vi "Actor Core.vi"(8 "error in":errorcluster caption="错误输入", 11 "上位机 in":refnum<class "上位机.lvclass"> caption="操作者输入") -> (0 "error out":errorcluster caption="错误输出", 3 "Actor out":refnum<class "Actor.lvclass"> caption="操作者输出")   [LabVIEW 2015, in "上位机.lvlib" / "上位机.lvclass"]
doc: "(<B>Filename</B>: Actor Framework.lvlib:Actor.lvclass:Actor Core.vi)\n\nReceives messages to the actor, reacts to them, and initiates any error handling that may shut the actor down.\n\nDescendant classes may override this VI to append parallel tasks for the actor to complete while it handles messages. Overrides use the Call Parent Method node."
uses:
  <vilib>/ActorFramework/Actor/Actor.lvclass
panel:
  in  "上位机标题":string
  out "接收内容":string
  in  "发送内容":string
  in  "发送":bool
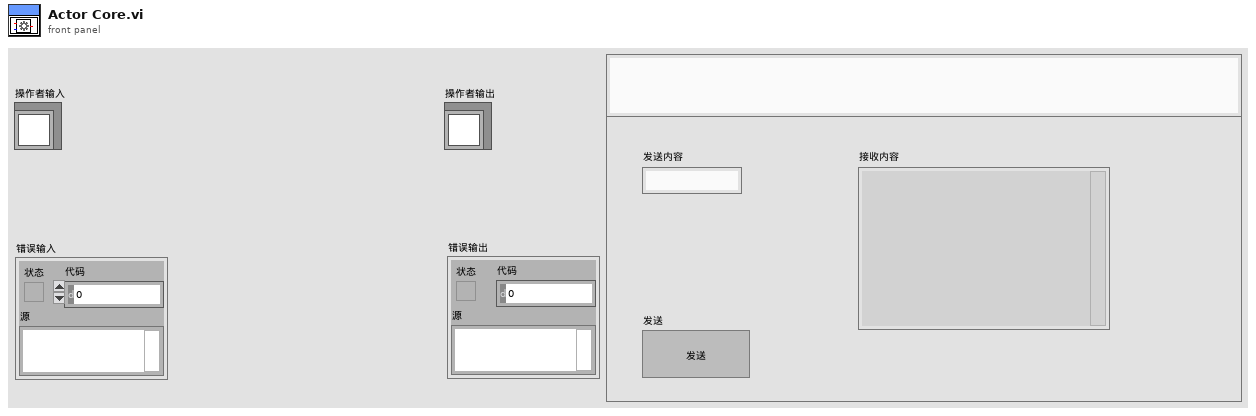
[diagram p1: front panel]
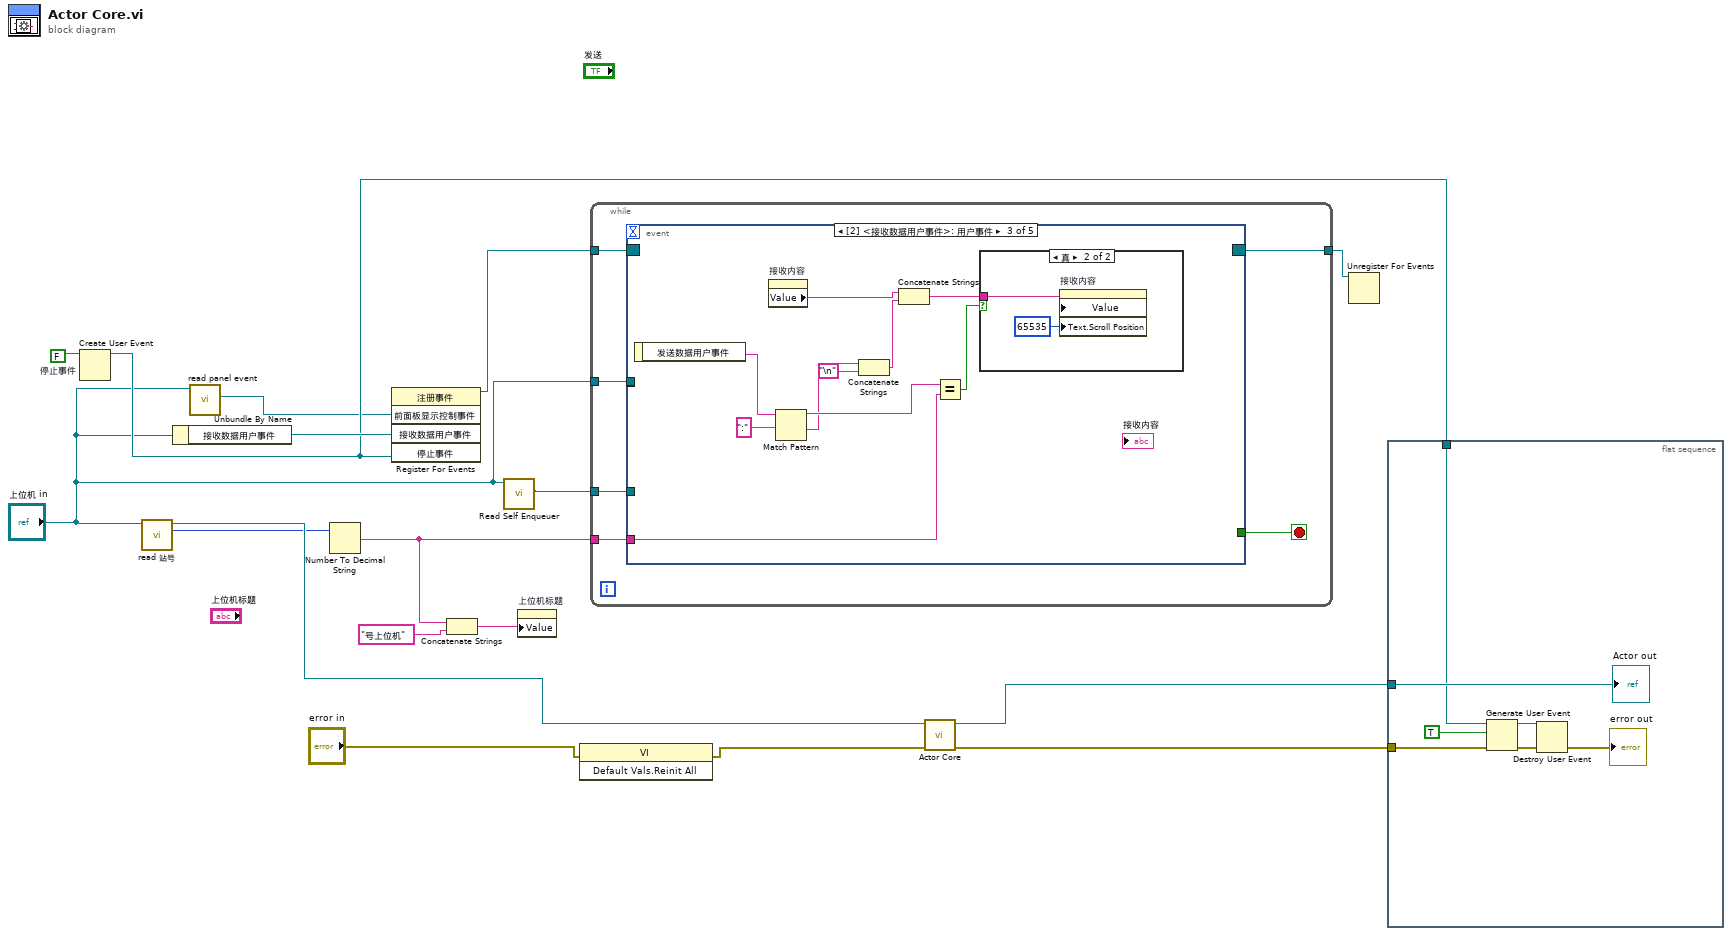
[diagram p0: block diagram]
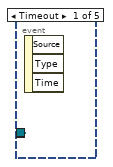
[diagram p2: hidden frame]
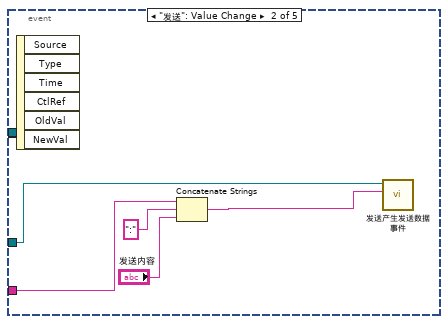
[diagram p3: hidden frame]
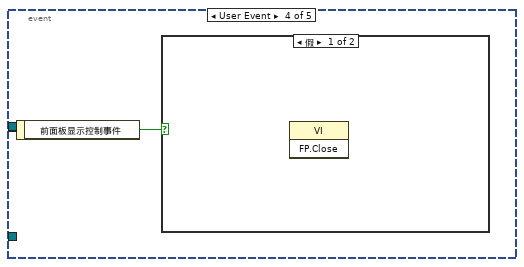
[diagram p5: hidden frame]
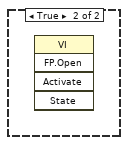
[diagram p6: hidden frame]
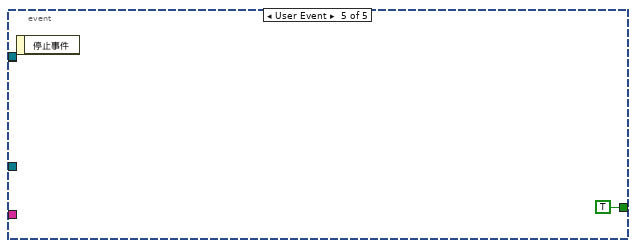
[diagram p7: hidden frame]
diagram:
  w9 = FALSE  # 停止事件
  n1 = Create User Event(user event datatype=w9) -> (user event=w8:refnum<user-event>)  [unwired: 1 in, 1 out]
  n2 = call "read 站号.vi"("上位机 输入"="上位机 in") -> ("站号"=w13:u8, "上位机 输出"=w14:refnum<class "上位机.lvclass">)  [unwired: 8 in, 1 out]
  n3 = Unbundle By Name("上位机 in") -> ("接收数据用户事件"=w11:refnum<user-event>)
  n4 = call "read panel event.vi"("前面板控制 输入"="上位机 in") -> ("前面板显示控制事件"=w3:refnum<user-event>)  [unwired: 8 in, 2 out]
  n5 = Number To Decimal String(number=w13) -> (decimal integer string=w6:string)  [unwired: 1 in]
  n6 = register-events(w3, w11, w8) -> (reference out=w16:refnum<event-registration>)  [unwired: 2 in, 1 out]
  n7 = Concatenate Strings(w6, "号上位机") -> (w5:string)
  n8 = call <vilib>:"Read Self Enqueuer.vi"("Actor"="上位机 in") -> ("Self Enqueuer"=w10:refnum<class "Message Enqueuer.lvclass">)  [unwired: 10 in]
  n9 = property on="上位机标题" class="Str"("Value"=w5) -> ()  [unwired: 2 in, 2 out]
  n10 = invoke class="VI" method="Default Vals.Reinit All"(error in="error in") -> (error out=w1:errorcluster)  [unwired: 2 in, 2 out]
  n11 = while {
    tunnel: w16 -> [w23]
    tunnel: [w22] -> w15
    tunnel: w10 -> [w21]
    tunnel: w6 -> [w20]
    tunnel: "上位机 in" -> [w18]
    stop <- w19 stop-if-true
    n12 = event shown="[2] <接收数据用户事件>: 用户事件" {
      selector: w23 -> [_ _ _ _ _]
      dyn-events: [_ _ _ _ _] -> w22
      timeout: _ -> [_ _ _ _ _]
      tunnel: w21 -> [_ w26 _ _ _]
      tunnel: w20 -> [_ w29 w33 _ _]
      tunnel: [_ _ _ _ TRUE] -> w19
      tunnel: [w24 _ _ _ _] -> _
      tunnel: w18 -> [w24 _ _ _ _]
      event Timeout {
        n13 = event-data() -> ()  [unwired: 1 in, 3 out]
      }
      event "发送": Value Change {
        n14 = event-data() -> ()  [unwired: 1 in, 6 out]
        n15 = Concatenate Strings(w29, ":" ("字符串"), "发送内容") -> (w25:string)
        n16 = call "发送产生发送数据事件.vi"("产生发送数据件数据"=w25, "Message Enqueuer"=w26) -> ()  [unwired: 8 in, 2 out]
      }
      event User Event {
        n17 = event-data() -> ("发送数据用户事件"=w35:string)  [unwired: 1 in]
        n18 = property on="接收内容" class="Str"() -> ("Value"=w38:string)  [unwired: 2 in, 2 out]
        n19 = Match Pattern(string=w35, regular expression=":" ("正则表达式")) -> (before substring=w32:string, after substring=w30:string)  [unwired: 1 in, 2 out]
        n20 = Concatenate Strings(w30, "\n") -> (w37:string)
        n21 = Concatenate Strings(w38, w37) -> (w36:string)
        n22 = Equal?(x=w32, y=w33) -> (x = y?=w31:bool)
        n23 = case shown="真" w31 {
          tunnel: w36 -> [_ w41]
          frame False {
          }
          frame True {
            n24 = property on="接收内容" class="Str"("Value"=w41, "Text.Scroll Position"=u32 65535 ("文本.滚动条位置")) -> ()  [unwired: 2 in, 2 out]
          }
        }
      }
      event User Event {
        n25 = event-data() -> ("前面板显示控制事件"=w42:bool)  [unwired: 1 in]
        n26 = case shown="假" w42 {
          frame False {
            n27 = invoke class="VI" method="FP.Close"() -> ()  [unwired: 3 in, 3 out]
          }
          frame True {
            n28 = invoke class="VI" method="FP.Open"() -> ()  [unwired: 5 in, 5 out]
          }
        }
      }
      event User Event {
        n29 = event-data() -> ()  [unwired: 1 in, 1 out]
      }
    }
  }
  n30 = call-parent "Actor Core.vi"("error in"=w1, "Actor in"=w14) -> ("error out"=w12:errorcluster, "Actor out"=w17:refnum<class "Actor.lvclass">)  [unwired: 8 in]
  n31 = Unregister For Events(event registration refnum=w15) -> ()  [unwired: 1 in, 1 out]
  n32 = flat-sequence {
    tunnel: w17 -> [w50]
    tunnel: w12 -> [w46]
    tunnel: w8 -> [w48]
    frame #0 {
      n33 = Generate User Event(user event=w48, event data cluster=TRUE, error in=w46) -> (user event out=w47:refnum<user-event>, error out=w45:errorcluster)  [unwired: 1 in]
      n34 = Destroy User Event(user event=w47, error in=w45) -> (error out=→"error out":errorcluster)
      "Actor out" <- w50
    }
  }
